vi "Create.vi"(8 "error in (no error)":errorcluster, 11 "FIFO size (10)":u32=10) -> (0 "error out":errorcluster, 3 "Plugin out":refnum<class "Plugin.lvclass">)   [LabVIEW 2016, in "Plugin.lvclass"]
uses:
  Plugin.lvclass
  Typdefs/Plugin FIFO Data.ctl
  Typdefs/Plugin Commands.ctl
  <vilib>/NI Veristand/VeriStand Data/Byte Buffer/Byte Buffer.Pointers.ctl
  Plugin.lvclass/Plugin.ctl
  Properties/Write Command FIFO.vi
  Properties/Write Response FIFO.vi
  <vilib>/NI Veristand/VeriStand Data/Byte Buffer/Byte Buffer.lvclass
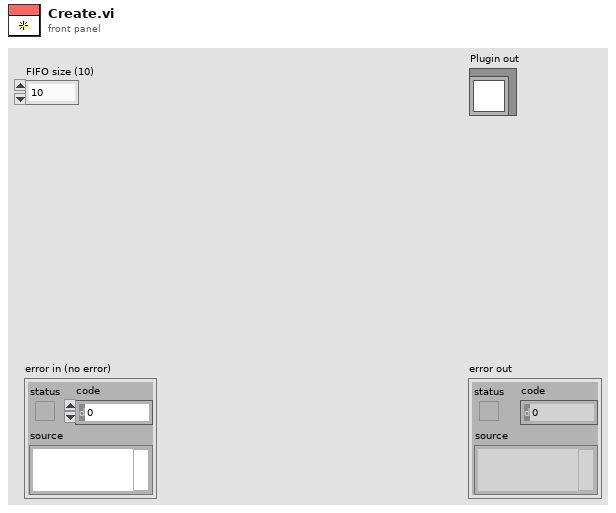
[diagram p1: front panel]
types:
  T1 = typedef "Plugin FIFO Data.ctl" = cluster{"Command":T2, "Byte Buffer pointers":T3}
  T2 = typedef "Plugin Commands.ctl" = enum16{"Process Buffer", "Shutdown"}
  T3 = typedef "VeriStand Data.lvlib/Byte Buffer.lvclass/Byte Buffer.Pointers.ctl" = cluster{"buffer data ptr":u64, "buffer size ptr":u64, "byte order ptr":u64}
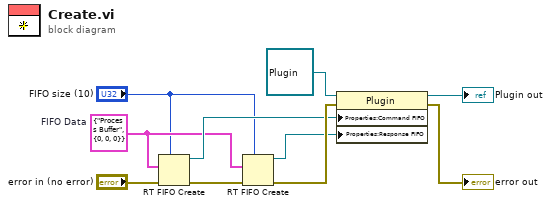
[diagram p0: block diagram]
diagram:
  w6 = T1 {"Command"=enum."Process Buffer", "Byte Buffer pointers"={"buffer data ptr"=0, "buffer size ptr"=0, "byte order ptr"=0}}  # FIFO Data
  n1 = RT FIFO Create(1:w6, 3:"error in (no error)", 4:"FIFO size (10)") -> (8:w8:refnum<k33>, 11:w5:errorcluster)  [unwired: 5 in, 1 out]
  n2 = RT FIFO Create(1:w6, 3:w5, 4:"FIFO size (10)") -> (8:w4:refnum<k33>, 11:w10:errorcluster)  [unwired: 5 in, 1 out]
  n3 = property class="Plugin"(reference=refnum<class "Plugin.lvclass"> refnum ("Plugin"), error in=w10, "Properties:Command FIFO"=w8, "Properties:Response FIFO"=w4) -> (reference out=→"Plugin out":refnum<class "Plugin.lvclass">, error out=→"error out":errorcluster)
